vi "nanocal -- nuclear schottky fit V7.vi"() -> ()   [LabVIEW 2021] (continued)
   ,  \"τC\" -> 0.002285007383   ,  \"κ0\" -> 0.000000022392   ,  \"mm1\" -> 0.000029550397   ,  \"mm2\" -> 0.012249707235   ,  \"mm3\" -> 0.037312700617   ,  \"T\" -> 3.100000000000   ,  \"B\" -> 4.000000000000   ,  \"θ\" -> 90.000000000000   ,  \"Reoff\" -> -175510.204081632662   ,  \"Imoff\" -> 0.000000000000   ,  \"στ1\" -> 0.000595847504   ,  \"στS\" -> 0.000046124245   ,  \"στN\" -> 0.000000091796    |>   , \n\"IDS0609_220610_RAW_cal__sam_\" ->   <|    \"ζ\" -> 0.000000000000   ,  \"τ1\" -> 0.000000000000   ,  \"τS\" -> 0.000000000000   ,  \"τN\" -> 0.000000000000   ,  \"τC\" -> 0.000000000000   ,  \"κ0\" -> 0.000000000000   ,  \"mm1\" -> 0.000000000000   ,  \"mm2\" -> 0.000000000000   ,  \"mm3\" -> 0.000000000000   ,  \"T\" -> 3.100000000000   ,  \"B\" -> 4.000000000000   ,  \"θ\" -> 90.000000000000   ,  \"Reoff\" -> 0.000000000000   ,  \"Imoff\" -> 0.000000000000   ,  \"στ1\" -> 0.000000000000   ,  \"στS\" -> 0.000000000000   ,  \"στN\" -> 0.000000000000    |>   , \n\"IDS0610_220610_RAW_cal__ref_\" ->   <|    \"ζ\" -> 0.017289416692   ,  \"τ1\" -> 0.037297104830   ,  \"τS\" -> 0.006044321671   ,  \"τN\" -> 0.000001504072   ,  \"τC\" -> 0.001946264025   ,  \"κ0\" -> 0.000000055145   ,  \"mm1\" -> 0.000025203584   ,  \"mm2\" -> 0.008069462881   ,  \"mm3\" -> 0.037299056933   ,  \"T\" -> 5.700000000000   ,  \"B\" -> 4.000000000000   ,  \"θ\" -> 90.000000000000   ,  \"Reoff\" -> -61224.489795918343   ,  \"Imoff\" -> 0.000000000000   ,  \"στ1\" -> 0.009662236305   ,  \"στS\" -> 0.002526126048   ,  \"στN\" -> 0.000001649991    |>   , \n\"IDS0610_220610_RAW_cal__sam_\" ->   <|    \"ζ\" -> 0.000000000000   ,  \"τ1\" -> 0.000000000000   ,  \"τS\" -> 0.000000000000   ,  \"τN\" -> 0.000000000000   ,  \"τC\" -> 0.000000000000   ,  \"κ0\" -> 0.000000000000   ,  \"mm1\" -> 0.000000000000   ,  \"mm2\" -> 0.000000000000   ,  \"mm3\" -> 0.000000000000   ,  \"T\" -> 5.700000000000   ,  \"B\" -> 4.000000000000   ,  \"θ\" -> 90.000000000000   ,  \"Reoff\" -> 0.000000000000   ,  \"Imoff\" -> 0.000000000000   ,  \"στ1\" -> 0.000000000000   ,  \"στS\" -> 0.000000000000   ,  \"στN\" -> 0.000000000000    |>   , \n\"IDS0612_220610_RAW_cal__ref_\" ->   <|    \"ζ\" -> 0.027806171987   ,  \"τ1\" -> 0.017638558844   ,  \"τS\" -> 0.022454693159   ,  \"τN\" -> 0.000230606872   ,  \"τC\" -> 0.002790453039   ,  \"κ0\" -> 0.000000005094   ,  \"mm1\" -> 0.000067525510   ,  \"mm2\" -> 0.017167524250   ,  \"mm3\" -> 0.026510053509   ,  \"T\" -> 0.820000000000   ,  \"B\" -> 5.000000000000   ,  \"θ\" -> 90.000000000000   ,  \"Reoff\" -> -885714.285714285680   ,  \"Imoff\" -> 0.000000000000   ,  \"στ1\" -> 0.001146653541   ,  \"στS\" -> 0.000179915023   ,  \"στN\" -> 0.000004482288    |>   , \n\"IDS0612_220610_RAW_cal__sam_\" ->   <|    \"ζ\" -> 0.000000000000   ,  \"τ1\" -> 0.000000000000   ,  \"τS\" -> 0.000000000000   ,  \"τN\" -> 0.000000000000   ,  \"τC\" -> 0.000000000000   ,  \"κ0\" -> 0.000000000000   ,  \"mm1\" -> 0.000000000000   ,  \"mm2\" -> 0.000000000000   ,  \"mm3\" -> 0.000000000000   ,  \"T\" -> 0.820000000000   ,  \"B\" -> 5.000000000000   ,  \"θ\" -> 90.000000000000   ,  \"Reoff\" -> 0.000000000000   ,  \"Imoff\" -> 0.000000000000   ,  \"στ1\" -> 0.000000000000   ,  \"στS\" -> 0.000000000000   ,  \"στN\" -> 0.000000000000    |>   , \n\"IDS0613_220610_RAW_cal__ref_\" ->   <|    \"ζ\" -> 0.023917075048   ,  \"τ1\" -> 0.017613265802   ,  \"τS\" -> 0.018183300032   ,  \"τN\" -> 0.000148874581   ,  \"τC\" -> 0.002629507092   ,  \"κ0\" -> 0.000000007146   ,  \"mm1\" -> 0.000053956796   ,  \"mm2\" -> 0.016996296873   ,  \"mm3\" -> 0.021963145834   ,  \"T\" -> 1.120000000000   ,  \"B\" -> 5.000000000000   ,  \"θ\" -> 90.000000000000   ,  \"Reoff\" -> -877551.020408163311   ,  \"Imoff\" -> 0.000000000000   ,  \"στ1\" -> 0.001189746119   ,  \"στS\" -> 0.000158276904   ,  \"στN\" -> 0.000002453686    |>   , \n\"IDS0613_220610_RAW_cal__sam_\" ->   <|    \"ζ\" -> 0.000000000000   ,  \"τ1\" -> 0.000000000000   ,  \"τS\" -> 0.000000000000   ,  \"τN\" -> 0.000000000000   ,  \"τC\" -> 0.000000000000   ,  \"κ0\" -> 0.000000000000   ,  \"mm1\" -> 0.000000000000   ,  \"mm2\" -> 0.000000000000   ,  \"mm3\" -> 0.000000000000   ,  \"T\" -> 1.120000000000   ,  \"B\" -> 5.000000000000   ,  \"θ\" -> 90.000000000000   ,  \"Reoff\" -> 0.000000000000   ,  \"Imoff\" -> 0.000000000000   ,  \"στ1\" -> 0.000000000000   ,  \"στS\" -> 0.000000000000   ,  \"στN\" -> 0.000000000000    |>   , \n\"IDS0614_220610_RAW_cal__ref_\" ->   <|    \"ζ\" -> 0.017909358082   ,  \"τ1\" -> 0.017480687226   ,  \"τS\" -> 0.012860329043   ,  \"τN\" -> 0.000077799463   ,  \"τC\" -> 0.003015067786   ,  \"κ0\" -> 0.000000012573   ,  \"mm1\" -> 0.000043232989   ,  \"mm2\" -> 0.015457741040   ,  \"mm3\" -> 0.018164623065   ,  \"T\" -> 1.900000000000   ,  \"B\" -> 5.000000000000   ,  \"θ\" -> 90.000000000000   ,  \"Reoff\" -> -330612.244897959171   ,  \"Imoff\" -> 0.000000000000   ,  \"στ1\" -> 0.000912905894   ,  \"στS\" -> 0.000088716304   ,  \"στN\" -> 0.000002113548    |>   , \n\"IDS0614_220610_RAW_cal__sam_\" ->   <|    \"ζ\" -> 0.000000000000   ,  \"τ1\" -> 0.000000000000   ,  \"τS\" -> 0.000000000000   ,  \"τN\" -> 0.000000000000   ,  \"τC\" -> 0.000000000000   ,  \"κ0\" -> 0.000000000000   ,  \"mm1\" -> 0.000000000000   ,  \"mm2\" -> 0.000000000000   ,  \"mm3\" -> 0.000000000000   ,  \"T\" -> 1.900000000000   ,  \"B\" -> 5.000000000000   ,  \"θ\" -> 90.000000000000   ,  \"Reoff\" -> 0.000000000000   ,  \"Imoff\" -> 0.000000000000   ,  \"στ1\" -> 0.000000000000   ,  \"στS\" -> 0.000000000000   ,  \"στN\" -> 0.000000000000    |>   , \n\"IDS0615_220610_RAW_cal__ref_\" ->   <|    \"ζ\" -> 0.018184973350   ,  \"τ1\" -> 0.017408880913   ,  \"τS\" -> 0.009354983655   ,  \"τN\" -> 0.000026355523   ,  \"τC\" -> 0.002778499813   ,  \"κ0\" -> 0.000000022360   ,  \"mm1\" -> 0.000038538571   ,  \"mm2\" -> 0.012202232609   ,  \"mm3\" -> 0.017498548126   ,  \"T\" -> 3.100000000000   ,  \"B\" -> 5.000000000000   ,  \"θ\" -> 90.000000000000   ,  \"Reoff\" -> -191836.734693877515   ,  \"Imoff\" -> 0.000000000000   ,  \"στ1\" -> 0.001312365409   ,  \"στS\" -> 0.000063057161   ,  \"στN\" -> 0.000000988894    |>   , \n\"IDS0615_220610_RAW_cal__sam_\" ->   <|    \"ζ\" -> 0.000000000000   ,  \"τ1\" -> 0.000000000000   ,  \"τS\" -> 0.000000000000   ,  \"τN\" -> 0.000000000000   ,  \"τC\" -> 0.000000000000   ,  \"κ0\" -> 0.000000000000   ,  \"mm1\" -> 0.000000000000   ,  \"mm2\" -> 0.000000000000   ,  \"mm3\" -> 0.000000000000   ,  \"T\" -> 3.100000000000   ,  \"B\" -> 5.000000000000   ,  \"θ\" -> 90.000000000000   ,  \"Reoff\" -> 0.000000000000   ,  \"Imoff\" -> 0.000000000000   ,  \"στ1\" -> 0.000000000000   ,  \"στS\" -> 0.000000000000   ,  \"στN\" -> 0.000000000000    |>   , \n\"IDS0616_220610_RAW_cal__ref_\" ->   <|    \"ζ\" -> 0.021580744060   ,  \"τ1\" -> 0.018863304594   ,  \"τS\" -> 0.006040479317   ,  \"τN\" -> 0.000014968890   ,  \"τC\" -> 0.001981910818   ,  \"κ0\" -> 0.000000054950   ,  \"mm1\" -> 0.000031813796   ,  \"mm2\" -> 0.008109417181   ,  \"mm3\" -> 0.018890113720   ,  \"T\" -> 5.700000000000   ,  \"B\" -> 5.000000000000   ,  \"θ\" -> 90.000000000000   ,  \"Reoff\" -> -102040.816326530650   ,  \"Imoff\" -> 0.000000000000   ,  \"στ1\" -> 0.003832459400   ,  \"στS\" -> 0.000063285444   ,  \"στN\" -> 0.000001437164    |>   , \n\"IDS0616_220610_RAW_cal__sam_\" ->   <|    \"ζ\" -> 0.000000000000   ,  \"τ1\" -> 0.000000000000   ,  \"τS\" -> 0.000000000000   ,  \"τN\" -> 0.000000000000   ,  \"τC\" -> 0.000000000000   ,  \"κ0\" -> 0.000000000000   ,  \"mm1\" -> 0.000000000000   ,  \"mm2\" -> 0.000000000000   ,  \"mm3\" -> 0.000000000000   ,  \"T\" -> 5.700000000000   ,  \"B\" -> 5.000000000000   ,  \"θ\" -> 90.000000000000   ,  \"Reoff\" -> 0.000000000000   ,  \"Imoff\" -> 0.000000000000   ,  \"στ1\" -> 0.000000000000   ,  \"στS\" -> 0.000000000000   ,  \"στN\" -> 0.000000000000    |>   , \n\"IDS0618_220610_RAW_cal__ref_\" ->   <|    \"ζ\" -> 0.038971550776   ,  \"τ1\" -> 0.018146117143   ,  \"τS\" -> 0.027126639064   ,  \"τN\" -> 0.001095165707   ,  \"τC\" -> 0.001889759396   ,  \"κ0\" -> 0.000000003734   ,  \"mm1\" -> 0.000066576943   ,  \"mm2\" -> 0.016715518022   ,  \"mm3\" -> 0.032575433843   ,  \"T\" -> 0.620000000000   ,  \"B\" -> 8.000000000000   ,  \"θ\" -> 90.000000000000   ,  \"Reoff\" -> -2648979.591836734680   ,  \"Imoff\" -> 0.000000000000   ,  \"στ1\" -> 0.003517417724   ,  \"στS\" -> 0.000462948011   ,  \"στN\" -> 0.000116737620    |>   , \n\"IDS0618_220610_RAW_cal__sam_\" ->   <|    \"ζ\" -> 0.000000000000   ,  \"τ1\" -> 0.000000000000   ,  \"τS\" -> 0.000000000000   ,  \"τN\" -> 0.000000000000   ,  \"τC\" -> 0.000000000000   ,  \"κ0\" -> 0.000000000000   ,  \"mm1\" -> 0.000000000000   ,  \"mm2\" -> 0.000000000000   ,  \"mm3\" -> 0.000000000000   ,  \"T\" -> 0.620000000000   ,  \"B\" -> 8.000000000000   ,  \"θ\" -> 90.000000000000   ,  \"Reoff\" -> 0.000000000000   ,  \"Imoff\" -> 0.000000000000   ,  \"στ1\" -> 0.000000000000   ,  \"στS\" -> 0.000000000000   ,  \"στN\" -> 0.000000000000    |>   , \n\"IDS0619_220610_RAW_cal__ref_\" ->   <|    \"ζ\" -> 0.024009223885   ,  \"τ1\" -> 0.018709750105   ,  \"τS\" -> 0.019196212155   ,  \"τN\" -> 0.000222399775   ,  \"τC\" -> 0.002606828702   ,  \"κ0\" -> 0.000000007177   ,  \"mm1\" -> 0.000054095260   ,  \"mm2\" -> 0.017792742522   ,  \"mm3\" -> 0.023354578757   ,  \"T\" -> 1.120000000000   ,  \"B\" -> 8.000000000000   ,  \"θ\" -> 90.000000000000   ,  \"Reoff\" -> -885714.285714285447   ,  \"Imoff\" -> 0.000000000000   ,  \"στ1\" -> 0.006664321445   ,  \"στS\" -> 0.000168480211   ,  \"στN\" -> 0.000061133182    |>   , \n\"IDS0619_220610_RAW_cal__sam_\" ->   <|    \"ζ\" -> 0.000000000000   ,  \"τ1\" -> 0.000000000000   ,  \"τS\" -> 0.000000000000   ,  \"τN\" -> 0.000000000000   ,  \"τC\" -> 0.000000000000   ,  \"κ0\" -> 0.000000000000   ,  \"mm1\" -> 0.000000000000   ,  \"mm2\" -> 0.000000000000   ,  \"mm3\" -> 0.000000000000   ,  \"T\" -> 1.120000000000   ,  \"B\" -> 8.000000000000   ,  \"θ\" -> 90.000000000000   ,  \"Reoff\" -> 0.000000000000   ,  \"Imoff\" -> 0.000000000000   ,  \"στ1\" -> 0.000000000000   ,  \"στS\" -> 0.000000000000   ,  \"στN\" -> 0.000000000000    |>   , \n\"IDS0620_220610_RAW_cal__ref_\" ->   <|    \"ζ\" -> 0.017708509932   ,  \"τ1\" -> 0.018998736540   ,  \"τS\" -> 0.013522892780   ,  \"τN\" -> 0.000111412007   ,  \"τC\" -> 0.002986591079   ,  \"κ0\" -> 0.000000012545   ,  \"mm1\" -> 0.000042810446   ,  \"mm2\" -> 0.016081465537   ,  \"mm3\" -> 0.019736799645   ,  \"T\" -> 1.900000000000   ,  \"B\" -> 8.000000000000   ,  \"θ\" -> 90.000000000000   ,  \"Reoff\" -> -322448.979591836221   ,  \"Imoff\" -> 0.000000000000   ,  \"στ1\" -> 0.002489183106   ,  \"στS\" -> 0.000085913917   ,  \"στN\" -> 0.000005325276    |>   , \n\"IDS0620_220610_RAW_cal__sam_\" ->   <|    \"ζ\" -> 0.000000000000   ,  \"τ1\" -> 0.000000000000   ,  \"τS\" -> 0.000000000000   ,  \"τN\" -> 0.000000000000   ,  \"τC\" -> 0.000000000000   ,  \"κ0\" -> 0.000000000000   ,  \"mm1\" -> 0.000000000000   ,  \"mm2\" -> 0.000000000000   ,  \"mm3\" -> 0.000000000000   ,  \"T\" -> 1.900000000000   ,  \"B\" -> 8.000000000000   ,  \"θ\" -> 90.000000000000   ,  \"Reoff\" -> 0.000000000000   ,  \"Imoff\" -> 0.000000000000   ,  \"στ1\" -> 0.000000000000   ,  \"στS\" -> 0.000000000000   ,  \"στN\" -> 0.000000000000    |>   , \n\"IDS0621_220610_RAW_cal__ref_\" ->   <|    \"ζ\" -> 0.017222795450   ,  \"τ1\" -> 0.018997433498   ,  \"τS\" -> 0.009525458339   ,  \"τN\" -> 0.000054927338   ,  \"τC\" -> 0.002829107724   ,  \"κ0\" -> 0.000000022378   ,  \"mm1\" -> 0.000037185478   ,  \"mm2\" -> 0.012377068502   ,  \"mm3\" -> 0.019157673942   ,  \"T\" -> 3.100000000000   ,  \"B\" -> 8.000000000000   ,  \"θ\" -> 90.000000000000   ,  \"Reoff\" -> -175510.204081632662   ,  \"Imoff\" -> 0.000000000000   ,  \"στ1\" -> 0.000696462866   ,  \"στS\" -> 0.000049011590   ,  \"στN\" -> 0.000001187946    |>   , \n\"IDS0621_220610_RAW_cal__sam_\" ->   <|    \"ζ\" -> 0.000000000000   ,  \"τ1\" -> 0.000000000000   ,  \"τS\" -> 0.000000000000   ,  \"τN\" -> 0.000000000000   ,  \"τC\" -> 0.000000000000   ,  \"κ0\" -> 0.000000000000   ,  \"mm1\" -> 0.000000000000   ,  \"mm2\" -> 0.000000000000   ,  \"mm3\" -> 0.000000000000   ,  \"T\" -> 3.100000000000   ,  \"B\" -> 8.000000000000   ,  \"θ\" -> 90.000000000000   ,  \"Reoff\" -> 0.000000000000   ,  \"Imoff\" -> 0.000000000000   ,  \"στ1\" -> 0.000000000000   ,  \"στS\" -> 0.000000000000   ,  \"στN\" -> 0.000000000000    |>   , \n\"IDS0622_220610_RAW_cal__ref_\" ->   <|    \"ζ\" -> 0.018802685442   ,  \"τ1\" -> 0.018950322094   ,  \"τS\" -> 0.005932159284   ,  \"τN\" -> 0.000034155015   ,  \"τC\" -> 0.002206206702   ,  \"κ0\" -> 0.000000055128   ,  \"mm1\" -> 0.000029936955   ,  \"mm2\" -> 0.008193499351   ,  \"mm3\" -> 0.019011589520   ,  \"T\" -> 5.700000000000   ,  \"B\" -> 8.000000000000   ,  \"θ\" -> 90.000000000000   ,  \"Reoff\" -> -102040.816326530650   ,  \"Imoff\" -> 0.000000000000   ,  \"στ1\" -> 0.004091041448   ,  \"στS\" -> 0.000125318549   ,  \"στN\" -> 0.000002772070    |>   , \n\"IDS0622_220610_RAW_cal__sam_\" ->   <|    \"ζ\" -> 0.000000000000   ,  \"τ1\" -> 0.000000000000   ,  \"τS\" -> 0.000000000000   ,  \"τN\" -> 0.000000000000   ,  \"τC\" -> 0.000000000000   ,  \"κ0\" -> 0.000000000000   ,  \"mm1\" -> 0.000000000000   ,  \"mm2\" -> 0.000000000000   ,  \"mm3\" -> 0.000000000000   ,  \"T\" -> 5.700000000000   ,  \"B\" -> 8.000000000000   ,  \"θ\" -> 90.000000000000   ,  \"Reoff\" -> 0.000000000000   ,  \"Imoff\" -> 0.000000000000   ,  \"στ1\" -> 0.000000000000   ,  \"στS\" -> 0.000000000000   ,  \"στN\" -> 0.000000000000    |>   , \n\"IDS0624_220611_RAW_cal__ref_\" ->   <|    \"ζ\" -> 0.244976366635   ,  \"τ1\" -> 0.050051466083   ,  \"τS\" -> 0.039788798904   ,  \"τN\" -> 0.065150870551   ,  \"τC\" -> 0.000822741325   ,  \"κ0\" -> 0.000000000926   ,  \"mm1\" -> 0.000159743083   ,  \"mm2\" -> 0.015114289281   ,  \"mm3\" -> 0.166247583438   ,  \"T\" -> 0.200000000000   ,  \"B\" -> 10.000000000000   ,  \"θ\" -> 90.000000000000   ,  \"Reoff\" -> -42285714.285714268700   ,  \"Imoff\" -> 0.000000000000   ,  \"στ1\" -> 0.005729614410   ,  \"στS\" -> 0.001369922504   ,  \"στN\" -> 0.004796157705    |>   , \n\"IDS0624_220611_RAW_cal__sam_\" ->   <|    \"ζ\" -> 0.000000000000   ,  \"τ1\" -> 0.000000000000   ,  \"τS\" -> 0.000000000000   ,  \"τN\" -> 0.000000000000   ,  \"τC\" -> 0.000000000000   ,  \"κ0\" -> 0.000000000000   ,  \"mm1\" -> 0.000000000000   ,  \"mm2\" -> 0.000000000000   ,  \"mm3\" -> 0.000000000000   ,  \"T\" -> 0.200000000000   ,  \"B\" -> 10.000000000000   ,  \"θ\" -> 90.000000000000   ,  \"Reoff\" -> 0.000000000000   ,  \"Imoff\" -> 0.000000000000   ,  \"στ1\" -> 0.000000000000   ,  \"στS\" -> 0.000000000000   ,  \"στN\" -> 0.000000000000    |>   , \n\"IDS0625_220611_RAW_cal__ref_\" ->   <|    \"ζ\" -> 0.341296227559   ,  \"τ1\" -> 0.058698913640   ,  \"τS\" -> 0.044841481218   ,  \"τN\" -> 0.116701971458   ,  \"τC\" -> 0.000719554078   ,  \"κ0\" -> 0.000000000751   ,  \"mm1\" -> 0.000181455745   ,  \"mm2\" -> 0.013579301426   ,  \"mm3\" -> 0.262335334208   ,  \"T\" -> 0.170000000000   ,  \"B\" -> 10.000000000000   ,  \"θ\" -> 90.000000000000   ,  \"Reoff\" -> -78285714.285714283600   ,  \"Imoff\" -> 0.000000000000   ,  \"στ1\" -> 0.006389429330   ,  \"στS\" -> 0.001939647043   ,  \"στN\" -> 0.008335030843    |>   , \n\"IDS0625_220611_RAW_cal__sam_\" ->   <|    \"ζ\" -> 0.000000000000   ,  \"τ1\" -> 0.000000000000   ,  \"τS\" -> 0.000000000000   ,  \"τN\" -> 0.000000000000   ,  \"τC\" -> 0.000000000000   ,  \"κ0\" -> 0.000000000000   ,  \"mm1\" -> 0.000000000000   ,  \"mm2\" -> 0.000000000000   ,  \"mm3\" -> 0.000000000000   ,  \"T\" -> 0.170000000000   ,  \"B\" -> 10.000000000000   ,  \"θ\" -> 90.000000000000   ,  \"Reoff\" -> 0.000000000000   ,  \"Imoff\" -> 0.000000000000   ,  \"στ1\" -> 0.000000000000   ,  \"στS\" -> 0.000000000000   ,  \"στN\" -> 0.000000000000    |>   , \n\"IDS0626_220611_RAW_cal__ref_\" ->   <|    \"ζ\" -> 0.430834214152   ,  \"τ1\" -> 0.067490603382   ,  \"τS\" -> 0.050638360024   ,  \"τN\" -> 0.198477935722   ,  \"τC\" -> 0.000694762859   ,  \"κ0\" -> 0.000000000624   ,  \"mm1\" -> 0.000207784316   ,  \"mm2\" -> 0.011935695755   ,  \"mm3\" -> 0.412486005426   ,  \"T\" -> 0.150000000000   ,  \"B\" -> 10.000000000000   ,  \"θ\" -> 90.000000000000   ,  \"Reoff\" -> -115142857.142857134000   ,  \"Imoff\" -> 0.000000000000   ,  \"στ1\" -> 0.010786487534   ,  \"στS\" -> 0.003944576197   ,  \"στN\" -> 0.021401274735    |>   , \n\"IDS0626_220611_RAW_cal__sam_\" ->   <|    \"ζ\" -> 0.000000000000   ,  \"τ1\" -> 0.000000000000   ,  \"τS\" -> 0.000000000000   ,  \"τN\" -> 0.000000000000   ,  \"τC\" -> 0.000000000000   ,  \"κ0\" -> 0.000000000000   ,  \"mm1\" -> 0.000000000000   ,  \"mm2\" -> 0.000000000000   ,  \"mm3\" -> 0.000000000000   ,  \"T\" -> 0.150000000000   ,  \"B\" -> 10.000000000000   ,  \"θ\" -> 90.000000000000   ,  \"Reoff\" -> 0.000000000000   ,  \"Imoff\" -> 0.000000000000   ,  \"στ1\" -> 0.000000000000   ,  \"στS\" -> 0.000000000000   ,  \"στN\" -> 0.000000000000    |>   , \n\"IDS0627_220611_RAW_cal__ref_\" ->   <|    \"ζ\" -> 0.645741447314   ,  \"τ1\" -> 0.078535889200   ,  \"τS\" -> 0.057272545240   ,  \"τN\" -> 0.457037230896   ,  \"τC\" -> 0.000630659614   ,  \"κ0\" -> 0.000000000513   ,  \"mm1\" -> 0.000246422200   ,  \"mm2\" -> 0.008104140921   ,  \"mm3\" -> 0.917236901039   ,  \"T\" -> 0.120000000000   ,  \"B\" -> 10.000000000000   ,  \"θ\" -> 90.000000000000   ,  \"Reoff\" -> -140857142.857142866000   ,  \"Imoff\" -> 0.000000000000   ,  \"στ1\" -> 0.116986349472   ,  \"στS\" -> 0.055522403404   ,  \"στN\" -> 0.466381863920    |>   , \n\"IDS0627_220611_RAW_cal__sam_\" ->   <|    \"ζ\" -> 0.000000000000   ,  \"τ1\" -> 0.000000000000   ,  \"τS\" -> 0.000000000000   ,  \"τN\" -> 0.000000000000   ,  \"τC\" -> 0.000000000000   ,  \"κ0\" -> 0.000000000000   ,  \"mm1\" -> 0.000000000000   ,  \"mm2\" -> 0.000000000000   ,  \"mm3\" -> 0.000000000000   ,  \"T\" -> 0.120000000000   ,  \"B\" -> 10.000000000000   ,  \"θ\" -> 90.000000000000   ,  \"Reoff\" -> 0.000000000000   ,  \"Imoff\" -> 0.000000000000   ,  \"στ1\" -> 0.000000000000   ,  \"στS\" -> 0.000000000000   ,  \"στN\" -> 0.000000000000    |>   , \n\"IDS0628_220611_RAW_cal__ref_\" ->   <|    \"ζ\" -> 0.162802155917   ,  \"τ1\" -> 0.037674171056   ,  \"τS\" -> 0.033369422942   ,  \"τN\" -> 0.027695234809   ,  \"τC\" -> 0.000875515442   ,  \"κ0\" -> 0.000000001247   ,  \"mm1\" -> 0.000120233008   ,  \"mm2\" -> 0.015940588681   ,  \"mm3\" -> 0.093494980492   ,  \"T\" -> 0.250000000000   ,  \"B\" -> 10.000000000000   ,  \"θ\" -> 90.000000000000   ,  \"Reoff\" -> -23795918.367346938700   ,  \"Imoff\" -> 0.000000000000   ,  \"στ1\" -> 0.002046377961   ,  \"στS\" -> 0.000349741229   ,  \"στN\" -> 0.000860381660    |>   , \n\"IDS0628_220611_RAW_cal__sam_\" ->   <|    \"ζ\" -> 0.000000000000   ,  \"τ1\" -> 0.000000000000   ,  \"τS\" -> 0.000000000000   ,  \"τN\" -> 0.000000000000   ,  \"τC\" -> 0.000000000000   ,  \"κ0\" -> 0.000000000000   ,  \"mm1\" -> 0.000000000000   ,  \"mm2\" -> 0.000000000000   ,  \"mm3\" -> 0.000000000000   ,  \"T\" -> 0.250000000000   ,  \"B\" -> 10.000000000000   ,  \"θ\" -> 90.000000000000   ,  \"Reoff\" -> 0.000000000000   ,  \"Imoff\" -> 0.000000000000   ,  \"στ1\" -> 0.000000000000   ,  \"στS\" -> 0.000000000000   ,  \"στN\" -> 0.000000000000    |>   , \n\"IDS0629_220611_RAW_cal__ref_\" ->   <|    \"ζ\" -> 0.112190833427   ,  \"τ1\" -> 0.032183235509   ,  \"τS\" -> 0.030112114218   ,  \"τN\" -> 0.014171616737   ,  \"τC\" -> 0.000992984849   ,  \"κ0\" -> 0.000000001590   ,  \"mm1\" -> 0.000097554049   ,  \"mm2\" -> 0.016918790619   ,  \"mm3\" -> 0.065411835329   ,  \"T\" -> 0.300000000000   ,  \"B\" -> 10.000000000000   ,  \"θ\" -> 90.000000000000   ,  \"Reoff\" -> -13020408.163265310200   ,  \"Imoff\" -> 0.000000000000   ,  \"στ1\" -> 0.001718489505   ,  \"στS\" -> 0.000227881691   ,  \"στN\" -> 0.000458996023    |>   , \n\"IDS0629_220611_RAW_cal__sam_\" ->   <|    \"ζ\" -> 0.000000000000   ,  \"τ1\" -> 0.000000000000   ,  \"τS\" -> 0.000000000000   ,  \"τN\" -> 0.000000000000   ,  \"τC\" -> 0.000000000000   ,  \"κ0\" -> 0.000000000000   ,  \"mm1\" -> 0.000000000000   ,  \"mm2\" -> 0.000000000000   ,  \"mm3\" -> 0.000000000000   ,  \"T\" -> 0.300000000000   ,  \"B\" -> 10.000000000000   ,  \"θ\" -> 90.000000000000   ,  \"Reoff\" -> 0.000000000000   ,  \"Imoff\" -> 0.000000000000   ,  \"στ1\" -> 0.000000000000   ,  \"στS\" -> 0.000000000000   ,  \"στN\" -> 0.000000000000    |>   , \n\"IDS0630_220611_RAW_cal__ref_\" ->   <|    \"ζ\" -> 0.079968077159   ,  \"τ1\" -> 0.028703647271   ,  \"τS\" -> 0.027787521037   ,  \"τN\" -> 0.007458471541   ,  \"τC\" -> 0.001227018439   ,  \"κ0\" -> 0.000000002002   ,  \"mm1\" -> 0.000087530349   ,  \"mm2\" -> 0.017868351082   ,  \"mm3\" -> 0.050039331111   ,  \"T\" -> 0.360000000000   ,  \"B\" -> 10.000000000000   ,  \"θ\" -> 90.000000000000   ,  \"Reoff\" -> -6897959.183673471220   ,  \"Imoff\" -> 0.000000000000   ,  \"στ1\" -> 0.003375898444   ,  \"στS\" -> 0.000219600830   ,  \"στN\" -> 0.000437287365    |>   , \n\"IDS0630_220611_RAW_cal__sam_\" ->   <|    \"ζ\" -> 0.000000000000   ,  \"τ1\" -> 0.000000000000   ,  \"τS\" -> 0.000000000000   ,  \"τN\" -> 0.000000000000   ,  \"τC\" -> 0.000000000000   ,  \"κ0\" -> 0.000000000000   ,  \"mm1\" -> 0.000000000000   ,  \"mm2\" -> 0.000000000000   ,  \"mm3\" -> 0.000000000000   ,  \"T\" -> 0.360000000000   ,  \"B\" -> 10.000000000000   ,  \"θ\" -> 90.000000000000   ,  \"Reoff\" -> 0.000000000000   ,  \"Imoff\" -> 0.000000000000   ,  \"στ1\" -> 0.000000000000   ,  \"στS\" -> 0.000000000000   ,  \"στN\" -> 0.000000000000    |>   , \n\"IDS0631_220611_RAW_cal__ref_\" ->   <|    \"ζ\" -> 0.058778460979   ,  \"τ1\" -> 0.022115004364   ,  \"τS\" -> 0.025871969436   ,  \"τN\" -> 0.004788101555   ,  \"τC\" -> 0.001625064800   ,  \"κ0\" -> 0.000000002412   ,  \"mm1\" -> 0.000085411879   ,  \"mm2\" -> 0.015917070637   ,  \"mm3\" -> 0.040199809426   ,  \"T\" -> 0.420000000000   ,  \"B\" -> 10.000000000000   ,  \"θ\" -> 90.000000000000   ,  \"Reoff\" -> -2816326.530612244270   ,  \"Imoff\" -> 0.000000000000   ,  \"στ1\" -> 0.000587796710   ,  \"στS\" -> 0.000091605589   ,  \"στN\" -> 0.000126012019    |>   , \n\"IDS0631_220611_RAW_cal__sam_\" ->   <|    \"ζ\" -> 0.000000000000   ,  \"τ1\" -> 0.000000000000   ,  \"τS\" -> 0.000000000000   ,  \"τN\" -> 0.000000000000   ,  \"τC\" -> 0.000000000000   ,  \"κ0\" -> 0.000000000000   ,  \"mm1\" -> 0.000000000000   ,  \"mm2\" -> 0.000000000000   ,  \"mm3\" -> 0.000000000000   ,  \"T\" -> 0.420000000000   ,  \"B\" -> 10.000000000000   ,  \"θ\" -> 90.000000000000   ,  \"Reoff\" -> 0.000000000000   ,  \"Imoff\" -> 0.000000000000   ,  \"στ1\" -> 0.000000000000   ,  \"στS\" -> 0.000000000000   ,  \"στN\" -> 0.000000000000    |>   , \n\"IDS0632_220611_RAW_cal__ref_\" ->   <|    \"ζ\" -> 0.043876208110   ,  \"τ1\" -> 0.021478355659   ,  \"τS\" -> 0.024271049020   ,  \"τN\" -> 0.002270431826   ,  \"τC\" -> 0.001878964186   ,  \"κ0\" -> 0.000000003102   ,  \"mm1\" -> 0.000073722080   ,  \"mm2\" -> 0.017307979811   ,  \"mm3\" -> 0.033681638338   ,  \"T\" -> 0.520000000000   ,  \"B\" -> 10.000000000000   ,  \"θ\" -> 90.000000000000   ,  \"Reoff\" -> -1918367.346938774920   ,  \"Imoff\" -> 0.000000000000   ,  \"στ1\" -> 0.003137180042   ,  \"στS\" -> 0.000114620716   ,  \"στN\" -> 0.000177904413    |>   , \n\"IDS0632_220611_RAW_cal__sam_\" ->   <|    \"ζ\" -> 0.000000000000   ,  \"τ1\" -> 0.000000000000   ,  \"τS\" -> 0.000000000000   ,  \"τN\" -> 0.000000000000   ,  \"τC\" -> 0.000000000000   ,  \"κ0\" -> 0.000000000000   ,  \"mm1\" -> 0.000000000000   ,  \"mm2\" -> 0.000000000000   ,  \"mm3\" -> 0.000000000000   ,  \"T\" -> 0.520000000000   ,  \"B\" -> 10.000000000000   ,  \"θ\" -> 90.000000000000   ,  \"Reoff\" -> 0.000000000000   ,  \"Imoff\" -> 0.000000000000   ,  \"στ1\" -> 0.000000000000   ,  \"στS\" -> 0.000000000000   ,  \"στN\" -> 0.000000000000    |>   , \n\"IDS0633_220611_RAW_cal__ref_\" ->   <|    \"ζ\" -> 0.034677079160   ,  \"τ1\" -> 0.021718381386   ,  \"τS\" -> 0.023156430325   ,  \"τN\" -> 0.001263823282   ,  \"τC\" -> 0.002065959541   ,  \"κ0\" -> 0.000000003789   ,  \"mm1\" -> 0.000063900017   ,  \"mm2\" -> 0.018485786163   ,  \"mm3\" -> 0.030501731422   ,  \"T\" -> 0.620000000000   ,  \"B\" -> 10.000000000000   ,  \"θ\" -> 90.000000000000   ,  \"Reoff\" -> -1265306.122448978950   ,  \"Imoff\" -> 0.000000000000   ,  \"στ1\" -> 0.002060583109   ,  \"στS\" -> 0.000081647328   ,  \"στN\" -> 0.000097316031    |>   , \n\"IDS0633_220611_RAW_cal__sam_\" ->   <|    \"ζ\" -> 0.000000000000   ,  \"τ1\" -> 0.000000000000   ,  \"τS\" -> 0.000000000000   ,  \"τN\" -> 0.000000000000   ,  \"τC\" -> 0.000000000000   ,  \"κ0\" -> 0.000000000000   ,  \"mm1\" -> 0.000000000000   ,  \"mm2\" -> 0.000000000000   ,  \"mm3\" -> 0.000000000000   ,  \"T\" -> 0.620000000000   ,  \"B\" -> 10.000000000000   ,  \"θ\" -> 90.000000000000   ,  \"Reoff\" -> 0.000000000000   ,  \"Imoff\" -> 0.000000000000   ,  \"στ1\" -> 0.000000000000   ,  \"στS\" -> 0.000000000000   ,  \"στN\" -> 0.000000000000    |>   , \n\"IDS0634_220612_RAW_cal__ref_\" ->   <|    \"ζ\" -> 0.027036169383   ,  \"τ1\" -> 0.021733696350   ,  \"τS\" -> 0.021135918538   ,  \"τN\" -> 0.000553307170   ,  \"τC\" -> 0.002271656254   ,  \"κ0\" -> 0.000000005164   ,  \"mm1\" -> 0.000054257381   ,  \"mm2\" -> 0.019338329094   ,  \"mm3\" -> 0.026888385418   ,  \"T\" -> 0.820000000000   ,  \"B\" -> 10.000000000000   ,  \"θ\" -> 90.000000000000   ,  \"Reoff\" -> -938775.510204080491   ,  \"Imoff\" -> 0.000000000000   ,  \"στ1\" -> 0.001360200971   ,  \"στS\" -> 0.000123877284   ,  \"στN\" -> 0.000020166019    |>   , \n\"IDS0634_220612_RAW_cal__sam_\" ->   <|    \"ζ\" -> 0.000000000000   ,  \"τ1\" -> 0.000000000000   ,  \"τS\" -> 0.000000000000   ,  \"τN\" -> 0.000000000000   ,  \"τC\" -> 0.000000000000   ,  \"κ0\" -> 0.000000000000   ,  \"mm1\" -> 0.000000000000   ,  \"mm2\" -> 0.000000000000   ,  \"mm3\" -> 0.000000000000   ,  \"T\" -> 0.820000000000   ,  \"B\" -> 10.000000000000   ,  \"θ\" -> 90.000000000000   ,  \"Reoff\" -> 0.000000000000   ,  \"Imoff\" -> 0.000000000000   ,  \"στ1\" -> 0.000000000000   ,  \"στS\" -> 0.000000000000   ,  \"στN\" -> 0.000000000000    |>   , \n\"IDS0635_220612_RAW_cal__ref_\" ->   <|    \"ζ\" -> 0.022890647572   ,  \"τ1\" -> 0.021599440333   ,  \"τS\" -> 0.018784843036   ,  \"τN\" -> 0.000235286917   ,  \"τC\" -> 0.002353311778   ,  \"κ0\" -> 0.000000007245   ,  \"mm1\" -> 0.000047019578   ,  \"mm2\" -> 0.019399476842   ,  \"mm3\" -> 0.023961768735   ,  \"T\" -> 1.120000000000   ,  \"B\" -> 10.000000000000   ,  \"θ\" -> 90.000000000000   ,  \"Reoff\" -> -775510.204081632196   ,  \"Imoff\" -> 0.000000000000   ,  \"στ1\" -> 0.004256477992   ,  \"στS\" -> 0.000144718396   ,  \"στN\" -> 0.000029208339    |>   , \n\"IDS0635_220612_RAW_cal__sam_\" ->   <|    \"ζ\" -> 0.000000000000   ,  \"τ1\" -> 0.000000000000   ,  \"τS\" -> 0.000000000000   ,  \"τN\" -> 0.000000000000   ,  \"τC\" -> 0.000000000000   ,  \"κ0\" -> 0.000000000000   ,  \"mm1\" -> 0.000000000000   ,  \"mm2\" -> 0.000000000000   ,  \"mm3\" -> 0.000000000000   ,  \"T\" -> 1.120000000000   ,  \"B\" -> 10.000000000000   ,  \"θ\" -> 90.000000000000   ,  \"Reoff\" -> 0.000000000000   ,  \"Imoff\" -> 0.000000000000   ,  \"στ1\" -> 0.000000000000   ,  \"στS\" -> 0.000000000000   ,  \"στN\" -> 0.000000000000    |>   , \n\"IDS0636_220612_RAW_cal__ref_\" ->   <|    \"ζ\" -> 0.017457751366   ,  \"τ1\" -> 0.021556950502   ,  \"τS\" -> 0.013950093477   ,  \"τN\" -> 0.000069572481   ,  \"τC\" -> 0.002888715109   ,  \"κ0\" -> 0.000000012635   ,  \"mm1\" -> 0.000041283144   ,  \"mm2\" -> 0.016791744848   ,  \"mm3\" -> 0.021877055420   ,  \"T\" -> 1.900000000000   ,  \"B\" -> 10.000000000000   ,  \"θ\" -> 90.000000000000   ,  \"Reoff\" -> -285714.285714285448   ,  \"Imoff\" -> 0.000000000000   ,  \"στ1\" -> 0.002815711957   ,  \"στS\" -> 0.000085308545   ,  \"στN\" -> 0.000003509861    |>   , \n\"IDS0636_220612_RAW_cal__sam_\" ->   <|    \"ζ\" -> 0.000000000000   ,  \"τ1\" -> 0.000000000000   ,  \"τS\" -> 0.000000000000   ,  \"τN\" -> 0.000000000000   ,  \"τC\" -> 0.000000000000   ,  \"κ0\" -> 0.000000000000   ,  \"mm1\" -> 0.000000000000   ,  \"mm2\" -> 0.000000000000   ,  \"mm3\" -> 0.000000000000   ,  \"T\" -> 1.900000000000   ,  \"B\" -> 10.000000000000   ,  \"θ\" -> 90.000000000000   ,  \"Reoff\" -> 0.000000000000   ,  \"Imoff\" -> 0.000000000000   ,  \"στ1\" -> 0.000000000000   ,  \"στS\" -> 0.000000000000   ,  \"στN\" -> 0.000000000000    |>   , \n\"IDS0637_220612_RAW_cal__ref_\" ->   <|    \"ζ\" -> 0.017770105668   ,  \"τ1\" -> 0.021549186615   ,  \"τS\" -> 0.009965620739   ,  \"τN\" -> 0.000026194105   ,  \"τC\" -> 0.002636418134   ,  \"κ0\" -> 0.000000022540   ,  \"mm1\" -> 0.000036639875   ,  \"mm2\" -> 0.012704225708   ,  \"mm3\" -> 0.021614109615   ,  \"T\" -> 3.100000000000   ,  \"B\" -> 10.000000000000   ,  \"θ\" -> 90.000000000000   ,  \"Reoff\" -> -204081.632653061300   ,  \"Imoff\" -> 0.000000000000   ,  \"στ1\" -> 0.001593502412   ,  \"στS\" -> 0.000052874862   ,  \"στN\" -> 0.000000825186    |>   , \n\"IDS0637_220612_RAW_cal__sam_\" ->   <|    \"ζ\" -> 0.000000000000   ,  \"τ1\" -> 0.000000000000   ,  \"τS\" -> 0.000000000000   ,  \"τN\" -> 0.000000000000   ,  \"τC\" -> 0.000000000000   ,  \"κ0\" -> 0.000000000000   ,  \"mm1\" -> 0.000000000000   ,  \"mm2\" -> 0.000000000000   ,  \"mm3\" -> 0.000000000000   ,  \"T\" -> 3.100000000000   ,  \"B\" -> 10.000000000000   ,  \"θ\" -> 90.000000000000   ,  \"Reoff\" -> 0.000000000000   ,  \"Imoff\" -> 0.000000000000   ,  \"στ1\" -> 0.000000000000   ,  \"στS\" -> 0.000000000000   ,  \"στN\" -> 0.000000000000    |>   , \n\"IDS0638_220612_RAW_cal__ref_\" ->   <|    \"ζ\" -> 0.021698598791   ,  \"τ1\" -> 0.021496688345   ,  \"τS\" -> 0.006445256992   ,  \"τN\" -> 0.000009458169   ,  \"τC\" -> 0.001823286983   ,  \"κ0\" -> 0.000000055353   ,  \"mm1\" -> 0.000030436060   ,  \"mm2\" -> 0.008371803202   ,  \"mm3\" -> 0.021512509502   ,  \"T\" -> 5.700000000000   ,  \"B\" -> 10.000000000000   ,  \"θ\" -> 90.000000000000   ,  \"Reoff\" -> -122448.979591835290   ,  \"Imoff\" -> 0.000000000000   ,  \"στ1\" -> 0.002371185679   ,  \"στS\" -> 0.000866215672   ,  \"στN\" -> 0.000002921151    |>   , \n\"IDS0638_220612_RAW_cal__sam_\" ->   <|    \"ζ\" -> 0.000000000000   ,  \"τ1\" -> 0.000000000000   ,  \"τS\" -> 0.000000000000   ,  \"τN\" -> 0.000000000000   ,  \"τC\" -> 0.000000000000   ,  \"κ0\" -> 0.000000000000   ,  \"mm1\" -> 0.000000000000   ,  \"mm2\" -> 0.000000000000   ,  \"mm3\" -> 0.000000000000   ,  \"T\" -> 5.700000000000   ,  \"B\" -> 10.000000000000   ,  \"θ\" -> 90.000000000000   ,  \"Reoff\" -> 0.000000000000   ,  \"Imoff\" -> 0.000000000000   ,  \"στ1\" -> 0.000000000000   ,  \"στS\" -> 0.000000000000   ,  \"στN\" -> 0.000000000000    |>   , \n\"IDS0640_220612_RAW_cal__ref_\" ->   <|    \"ζ\" -> 0.238834044855   ,  \"τ1\" -> 0.022929416344   ,  \"τS\" -> 0.072625980306   ,  \"τN\" -> 0.019844551932   ,  \"τC\" -> 0.000823612727   ,  \"κ0\" -> 0.000000000936   ,  \"mm1\" -> 0.000157614859   ,  \"mm2\" -> 0.017180115008   ,  \"mm3\" -> 0.120970942686   ,  \"T\" -> 0.200000000000   ,  \"B\" -> 6.000000000000   ,  \"θ\" -> 90.000000000000   ,  \"Reoff\" -> -41673469.387755103400   ,  \"Imoff\" -> 0.000000000000   ,  \"στ1\" -> 0.013588787086   ,  \"στS\" -> 0.005909644069   ,  \"στN\" -> 0.005908317860    |>   , \n\"IDS0640_220612_RAW_cal__sam_\" ->   <|    \"ζ\" -> 0.000000000000   ,  \"τ1\" -> 0.000000000000   ,  \"τS\" -> 0.000000000000   ,  \"τN\" -> 0.000000000000   ,  \"τC\" -> 0.000000000000   ,  \"κ0\" -> 0.000000000000   ,  \"mm1\" -> 0.000000000000   ,  \"mm2\" -> 0.000000000000   ,  \"mm3\" -> 0.000000000000   ,  \"T\" -> 0.200000000000   ,  \"B\" -> 6.000000000000   ,  \"θ\" -> 90.000000000000   ,  \"Reoff\" -> 0.000000000000   ,  \"Imoff\" -> 0.000000000000   ,  \"στ1\" -> 0.000000000000   ,  \"στS\" -> 0.000000000000   ,  \"στN\" -> 0.000000000000    |>   , \n\"IDS0641_220612_RAW_cal__ref_\" ->   <|    \"ζ\" -> 0.337611684125   ,  \"τ1\" -> 0.024060482995   ,  \"τS\" -> 0.087442322349   ,  \"τN\" -> 0.039216913379   ,  \"τC\" -> 0.000779358096   ,  \"κ0\" -> 0.000000000742   ,  \"mm1\" -> 0.000195728848   ,  \"mm2\" -> 0.015872138171   ,  \"mm3\" -> 0.178192847684   ,  \"T\" -> 0.170000000000   ,  \"B\" -> 6.000000000000   ,  \"θ\" -> 90.000000000000   ,  \"Reoff\" -> -71142857.142857134400   ,  \"Imoff\" -> 0.000000000000   ,  \"στ1\" -> 0.018720628002   ,  \"στS\" -> 0.014050027266   ,  \"στN\" -> 0.015588773016    |>   , \n\"IDS0641_220612_RAW_cal__sam_\" ->   <|    \"ζ\" -> 0.000000000000   ,  \"τ1\" -> 0.000000000000   ,  \"τS\" -> 0.000000000000   ,  \"τN\" -> 0.000000000000   ,  \"τC\" -> 0.000000000000   ,  \"κ0\" -> 0.000000000000   ,  \"mm1\" -> 0.000000000000   ,  \"mm2\" -> 0.000000000000   ,  \"mm3\" -> 0.000000000000   ,  \"T\" -> 0.170000000000   ,  \"B\" -> 6.000000000000   ,  \"θ\" -> 90.000000000000   ,  \"Reoff\" -> 0.000000000000   ,  \"Imoff\" -> 0.000000000000   ,  \"στ1\" -> 0.000000000000   ,  \"στS\" -> 0.000000000000   ,  \"στN\" -> 0.000000000000    |>   , \n\"IDS0642_220612_RAW_cal__ref_\" ->   <|    \"ζ\" -> 0.425492131552   ,  \"τ1\" -> 0.026758245281   ,  \"τS\" -> 0.092876272141   ,  \"τN\" -> 0.068524187738   ,  \"τC\" -> 0.000712253308   ,  \"κ0\" -> 0.000000000634   ,  \"mm1\" -> 0.000211793649   ,  \"mm2\" -> 0.014653485868   ,  \"mm3\" -> 0.242680304659   ,  \"T\" -> 0.150000000000   ,  \"B\" -> 6.000000000000   ,  \"θ\" -> 90.000000000000   ,  \"Reoff\" -> -111171428.571428567000   ,  \"Imoff\" -> 0.000000000000   ,  \"στ1\" -> 0.016862211092   ,  \"στS\" -> 0.019282049224   ,  \"στN\" -> 0.022131638620    |>   , \n\"IDS0642_220612_RAW_cal__sam_\" ->   <|    \"ζ\" -> 0.000000000000   ,  \"τ1\" -> 0.000000000000   ,  \"τS\" -> 0.000000000000   ,  \"τN\" -> 0.000000000000   ,  \"τC\" -> 0.000000000000   ,  \"κ0\" -> 0.000000000000   ,  \"mm1\" -> 0.000000000000   ,  \"mm2\" -> 0.000000000000   ,  \"mm3\" -> 0.000000000000   ,  \"T\" -> 0.150000000000   ,  \"B\" -> 6.000000000000   ,  \"θ\" -> 90.000000000000   ,  \"Reoff\" -> 0.000000000000   ,  \"Imoff\" -> 0.000000000000   ,  \"στ1\" -> 0.000000000000   ,  \"στS\" -> 0.000000000000   ,  \"στN\" -> 0.000000000000    |>   , \n\"IDS0643_220612_RAW_cal__ref_\" ->   <|    \"ζ\" -> 0.645665826507   ,  \"τ1\" -> 0.033591555956   ,  \"τS\" -> 0.115598019979   ,  \"τN\" -> 0.189817561833   ,  \"τC\" -> 0.000794602780   ,  \"κ0\" -> 0.000000000472   ,  \"mm1\" -> 0.000310954135   ,  \"mm2\" -> 0.012215752320   ,  \"mm3\" -> 0.524471438152   ,  \"T\" -> 0.120000000000   ,  \"B\" -> 6.000000000000   ,  \"θ\" -> 90.000000000000   ,  \"Reoff\" -> -174187755.102040827000   ,  \"Imoff\" -> 0.000000000000   ,  \"στ1\" -> 0.039640874529   ,  \"στS\" -> 0.065981071320   ,  \"στN\" -> 0.095740947662    |>   , \n\"IDS0643_220612_RAW_cal__sam_\" ->   <|    \"ζ\" -> 0.000000000000   ,  \"τ1\" -> 0.000000000000   ,  \"τS\" -> 0.000000000000   ,  \"τN\" -> 0.000000000000   ,  \"τC\" -> 0.000000000000   ,  \"κ0\" -> 0.000000000000   ,  \"mm1\" -> 0.000000000000   ,  \"mm2\" -> 0.000000000000   ,  \"mm3\" -> 0.000000000000   ,  \"T\" -> 0.120000000000   ,  \"B\" -> 6.000000000000   ,  \"θ\" -> 90.000000000000   ,  \"Reoff\" -> 0.000000000000   ,  \"Imoff\" -> 0.000000000000   ,  \"στ1\" -> 0.000000000000   ,  \"στS\" -> 0.000000000000   ,  \"στN\" -> 0.000000000000    |>   , \n\"IDS0644_220612_RAW_cal__ref_\" ->   <|    \"ζ\" -> 0.159858410781   ,  \"τ1\" -> 0.020749494118   ,  \"τS\" -> 0.057576161881   ,  \"τN\" -> 0.009325169153   ,  \"τC\" -> 0.000895206146   ,  \"κ0\" -> 0.000000001246   ,  \"mm1\" -> 0.000121968889   ,  \"mm2\" -> 0.017087577763   ,  \"mm3\" -> 0.082031225104   ,  \"T\" -> 0.250000000000   ,  \"B\" -> 6.000000000000   ,  \"θ\" -> 90.000000000000   ,  \"Reoff\" -> -22730612.244897957900   ,  \"Imoff\" -> 0.000000000000   ,  \"στ1\" -> 0.009289428349   ,  \"στS\" -> 0.001695199729   ,  \"στN\" -> 0.001606279892    |>   , \n\"IDS0644_220612_RAW_cal__sam_\" ->   <|    \"ζ\" -> 0.000000000000   ,  \"τ1\" -> 0.000000000000   ,  \"τS\" -> 0.000000000000   ,  \"τN\" -> 0.000000000000   ,  \"τC\" -> 0.000000000000   ,  \"κ0\" -> 0.000000000000   ,  \"mm1\" -> 0.000000000000   ,  \"mm2\" -> 0.000000000000   ,  \"mm3\" -> 0.000000000000   ,  \"T\" -> 0.250000000000   ,  \"B\" -> 6.000000000000   ,  \"θ\" -> 90.000000000000   ,  \"Reoff\" -> 0.000000000000   ,  \"Imoff\" -> 0.000000000000   ,  \"στ1\" -> 0.000000000000   ,  \"στS\" -> 0.000000000000   ,  \"στN\" -> 0.000000000000    |>   , \n\"IDS0645_220612_RAW_cal__ref_\" ->   <|    \"ζ\" -> 0.118910946323   ,  \"τ1\" -> 0.019234304410   ,  \"τS\" -> 0.048411086474   ,  \"τN\" -> 0.005189783920   ,  \"τC\" -> 0.000853285420   ,  \"κ0\" -> 0.000000001572   ,  \"mm1\" -> 0.000089420282   ,  \"mm2\" -> 0.016698334707   ,  \"mm3\" -> 0.063274435457   ,  \"T\" -> 0.300000000000   ,  \"B\" -> 6.000000000000   ,  \"θ\" -> 90.000000000000   ,  \"Reoff\" -> -17734693.877551019200   ,  \"Imoff\" -> 0.000000000000   ,  \"στ1\" -> 0.002725843000   ,  \"στS\" -> 0.000632849867   ,  \"στN\" -> 0.000966939974    |>   , \n\"IDS0645_220612_RAW_cal__sam_\" ->   <|    \"ζ\" -> 0.000000000000   ,  \"τ1\" -> 0.000000000000   ,  \"τS\" -> 0.000000000000   ,  \"τN\" -> 0.000000000000   ,  \"τC\" -> 0.000000000000   ,  \"κ0\" -> 0.000000000000   ,  \"mm1\" -> 0.000000000000   ,  \"mm2\" -> 0.000000000000   ,  \"mm3\" -> 0.000000000000   ,  \"T\" -> 0.300000000000   ,  \"B\" -> 6.000000000000   ,  \"θ\" -> 90.000000000000   ,  \"Reoff\" -> 0.000000000000   ,  \"Imoff\" -> 0.000000000000   ,  \"στ1\" -> 0.000000000000   ,  \"στS\" -> 0.000000000000   ,  \"στN\" -> 0.000000000000    |>   , \n\"IDS0646_220612_RAW_cal__ref_\" ->   <|    \"ζ\" -> 0.082805615965   ,  \"τ1\" -> 0.018079378213   ,  \"τS\" -> 0.042371658617   ,  \"τN\" -> 0.002818805569   ,  \"τC\" -> 0.001126081150   ,  \"κ0\" -> 0.000000001982   ,  \"mm1\" -> 0.000084202319   ,  \"mm2\" -> 0.016434291092   ,  \"mm3\" -> 0.051619454361   ,  \"T\" -> 0.360000000000   ,  \"B\" -> 6.000000000000   ,  \"θ\" -> 90.000000000000   ,  \"Reoff\" -> -8204081.632653061300   ,  \"Imoff\" -> 0.000000000000   ,  \"στ1\" -> 0.000700707095   ,  \"στS\" -> 0.000241063025   ,  \"στN\" -> 0.000086776293    |>   , \n\"IDS0646_220612_RAW_cal__sam_\" ->   <|    \"ζ\" -> 0.000000000000   ,  \"τ1\" -> 0.000000000000   ,  \"τS\" -> 0.000000000000   ,  \"τN\" -> 0.000000000000   ,  \"τC\" -> 0.000000000000   ,  \"κ0\" -> 0.000000000000   ,  \"mm1\" -> 0.000000000000   ,  \"mm2\" -> 0.000000000000   ,  \"mm3\" -> 0.000000000000   ,  \"T\" -> 0.360000000000   ,  \"B\" -> 6.000000000000   ,  \"θ\" -> 90.000000000000   ,  \"Reoff\" -> 0.000000000000   ,  \"Imoff\" -> 0.000000000000   ,  \"στ1\" -> 0.000000000000   ,  \"στS\" -> 0.000000000000   ,  \"στN\" -> 0.000000000000    |>   , \n\"IDS0647_220612_RAW_cal__ref_\" ->   <|    \"ζ\" -> 0.061664152309   ,  \"τ1\" -> 0.016815828462   ,  \"τS\" -> 0.037558438894   ,  \"τN\" -> 0.001732753748   ,  \"τC\" -> 0.001485497584   ,  \"κ0\" -> 0.000000002383   ,  \"mm1\" -> 0.000083349881   ,  \"mm2\" -> 0.015688184969   ,  \"mm3\" -> 0.044243841925   ,  \"T\" -> 0.420000000000   ,  \"B\" -> 6.000000000000   ,  \"θ\" -> 90.000000000000   ,  \"Reoff\" -> -4297959.183673469350   ,  \"Imoff\" -> 0.000000000000   ,  \"στ1\" -> 0.001260209312   ,  \"στS\" -> 0.000277639724   ,  \"στN\" -> 0.000082943970    |>   , \n\"IDS0647_220612_RAW_cal__sam_\" ->   <|    \"ζ\" -> 0.000000000000   ,  \"τ1\" -> 0.000000000000   ,  \"τS\" -> 0.000000000000   ,  \"τN\" -> 0.000000000000   ,  \"τC\" -> 0.000000000000   ,  \"κ0\" -> 0.000000000000   ,  \"mm1\" -> 0.000000000000   ,  \"mm2\" -> 0.000000000000   ,  \"mm3\" -> 0.000000000000   ,  \"T\" -> 0.420000000000   ,  \"B\" -> 6.000000000000   ,  \"θ\" -> 90.000000000000   ,  \"Reoff\" -> 0.000000000000   ,  \"Imoff\" -> 0.000000000000   ,  \"στ1\" -> 0.000000000000   ,  \"στS\" -> 0.000000000000   ,  \"στN\" -> 0.000000000000    
